vi "DHE_DRV_write_memory.vi"(0 "fd":i32, 5 "type":string, 7 "address":i32, 9 "value":i32, 11 "error in (no error)":errorcluster) -> (4 "fd out":i32, 8 "return value":i32, 15 "error out":errorcluster)   [LabVIEW 2016]
doc: "This VI closes the I/O interface with the instrument."
uses:
  c/lib/libarcDHE.so
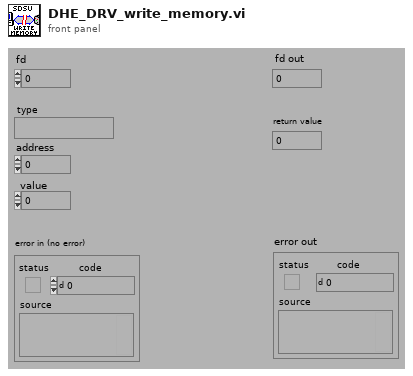
[diagram p1: front panel]
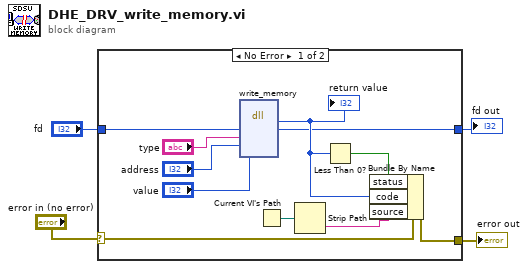
[diagram p0: block diagram]
diagram:
  n1 = case shown="No Error" "error in (no error)" {
    selector: "error in (no error)" -> [w5 w16]
    tunnel: [w11 w16] -> w4
    tunnel: "fd" -> [w7 w17]
    tunnel: [w6 w17] -> w2
    frame No Error {
      n2 = dll-call lib="home/simager/panview/PAN/Modules/SDSU/private/c/lib/libarcDHE.so" fn="write_memory"("fd"=w7, "type"="type", "address"="address", "value"="value") -> (w14:i32, "fd"=w6:i32)  [unwired: 6 in, 2 out]
      "return value" <- w14
      n3 = Current VI's Path() -> (path=w13:path)
      n4 = Strip Path(path=w13) -> (name=w12:string)  [unwired: 1 out]
      n5 = Less Than 0?(x=w14) -> (x < 0?=w15:bool)
      n6 = Bundle By Name(cluster=w5, "status"=w15, "code"=w14, "source"=w12) -> (w11:errorcluster)
    }
    frame Error {
    }
  }
  "error out" <- w4
  "fd out" <- w2
